vi "Set Position (SubVI).vi"(9 "Axis":i32, 10 "Position":dbl, 11 ".NET Refnum in":refnum<k24>) -> (0 "error out":errorcluster, 3 ".NET Refnum out":refnum<k24>)   [LabVIEW 2019, in "ESP301.lvlib"]
uses:
  ESP301.lvlib
  Newport.ESP301.CommandInterface
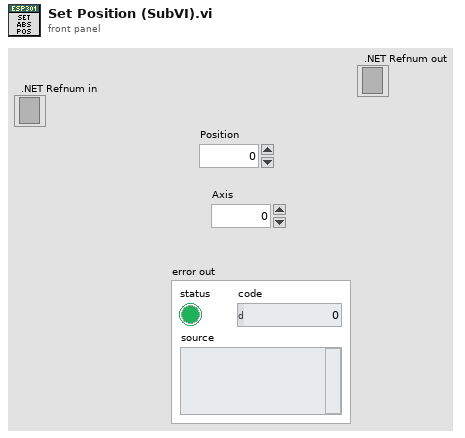
[diagram p1: front panel]
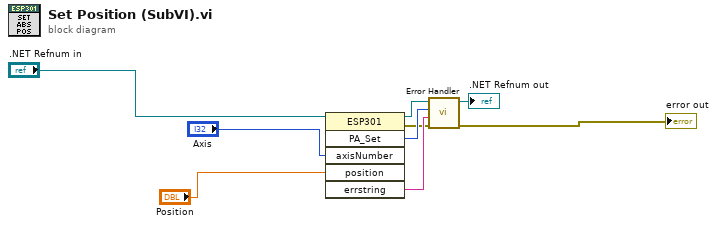
[diagram p0: block diagram]
diagram:
  n1 = invoke class="ESP301" method="PA_Set"(reference=".NET Refnum in", "axisNumber"="Axis", "position"="Position") -> (reference out=w7:refnum<k24>, error out=w5:errorcluster, "PA_Set"=w6:i32, "errstring"=w9:string)  [unwired: 3 in, 2 out]
  n2 = call "Error Handler.vi"("error in (no error)"=w5, "value"=w9, "OpenInstrument"=w6, ".NET Refnum in"=w7) -> ("error out"=→"error out":errorcluster, ".NET Refnum out"=→".NET Refnum out":refnum<k24>)  [unwired: 6 in]
